vi "Destroy.vi"(8 "Error In":errorcluster, 11 "reference in":refnum<class "VdAnalogInput_DAQmx.lvclass">) -> (0 "Error Out":errorcluster, 3 "reference out":refnum<class "VdAnalogInput_DAQmx.lvclass">)   [LabVIEW 2020, in "VdAnalogInput_DAQmx.lvclass"]
uses:
  VdAnalogInput_DAQmx.lvclass
  VdAnalogInput_DAQmx.lvclass/VdAnalogInput_DAQmx.ctl
  VdAnalogInput_class/VdAnalogInput.lvclass
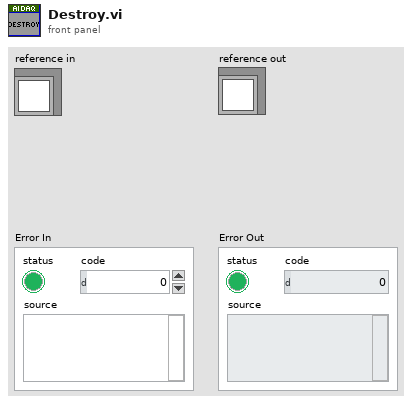
[diagram p1: front panel]
types:
  T1 = typedef "VdAnalogInput_DAQmx.lvclass/ObjectAttributes.ctl" = cluster{"task":refnum<k21>}
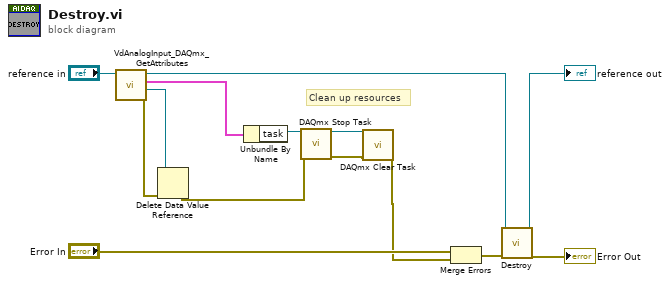
[diagram p0: block diagram]
diagram:
  # "Clean up resources"
  n1 = call "VdAnalogInput_DAQmx_GetAttributes.vi"("reference in"="reference in") -> ("error out"=w12:errorcluster, "DataRef"=w10:refnum<data-value>, "Data"=w6:T1, "reference out"=w11:refnum<class "VdAnalogInput_DAQmx.lvclass">)  [unwired: 7 in]
  n2 = Delete Data Value Reference(data value reference=w10, error in=w12) -> (error out=w2:errorcluster)  [unwired: 1 out]
  n3 = Unbundle By Name(w6) -> ("task"=w4:refnum<k21>)
  n4 = call <vilib>:"DAQmx Stop Task.vi"("task/channels in"=w4, "error in"=w2) -> ("task out"=w5:refnum<k21>, "error out"=w3:errorcluster)  [unwired: 12 in]
  n5 = call <vilib>:"DAQmx Clear Task.vi"("task in"=w5, "error in"=w3) -> ("error out"=w1:errorcluster)  [unwired: 13 in]
  n6 = Merge Errors("Error In", w1) -> (w14:errorcluster)
  n7 = call-parent "Destroy.vi"("Error In"=w14, "reference in"=w11) -> ("Error Out"=→"Error Out":errorcluster, "reference out"=→"reference out":refnum<class "VdAnalogInput_DAQmx.lvclass">)  [unwired: 8 in]
